vi "Ramp Wave Generator LUT.vi"(0 "frequency (periods/tick)":fxp<+,32,0>=0.0002500000409781933, 1 "reset":bool, 5 "phase offset (periods)":fxp<+,32,0>) -> (4 "saw out":i16)   [LabVIEW 2015]
doc: "Generates a point-by-point triangle wave using direct digital synthesis. The synthesis runs continuously from the top-level FPGA target clock to produce an accurate real-time frequency. Each execution of this VI returns the most recent sample produced by the underlying synthesis engine."
uses:
  <vilib>/rvi/Analysis/common/FxpNativeNode/niFpgaFxpNative.xnode
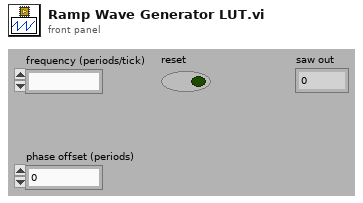
[diagram p1: front panel]
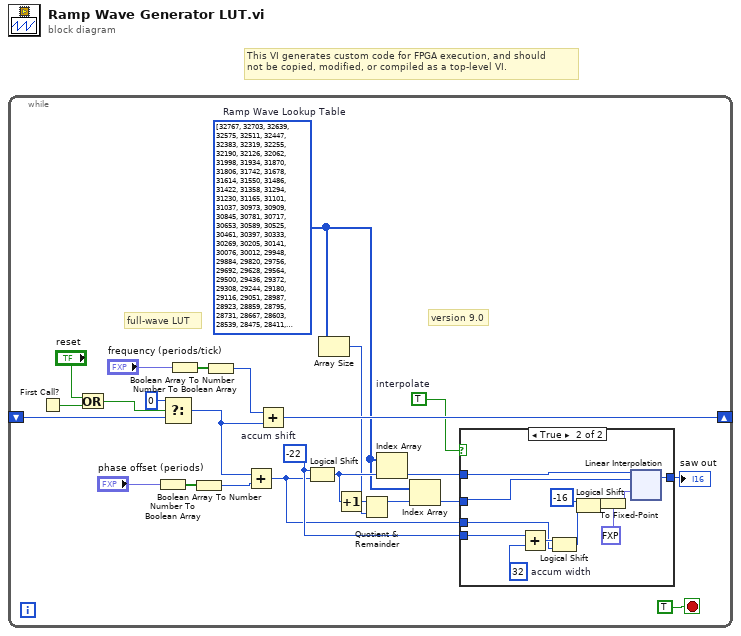
[diagram p0: block diagram]
diagram:
  # "This VI generates custom code for FPGA execution, and should\nnot be copied, modified, or compiled as a top-level VI."
  n1 = while {
    shift-right: [w24] -> _
    shift-left: _ -> [w17]
    stop <- TRUE stop-if-true
    w1 = i16[] [32767, 32703, 32639, 32575, 32511, 32447, 32383, 32319, 32255, 32190, 32126, 32062, 31998, 31934, 31870, 31806, 31742, 31678, 31614, 31550, 31486, 31422, 31358, 31294, 31230, 31165, 31101, 31037, 30973, 30909, 30845, 30781, 30717, 30653, 30589, 30525, 30461, 30397, 30333, 30269, 30205, 30141, 30076, 30012, 29948, 29884, 29820, 29756, 29692, 29628, 29564, 29500, 29436, 29372, 29308, 29244, 29180, 29116, 29051, 28987, 28923, 28859, 28795, 28731, 28667, 28603, 28539, 28475, 28411, 28347, 28283, 28219, 28155, 28091, 28027, 27962, 27898, 27834, 27770, 27706, 27642, 27578, 27514, 27450, 27386, 27322, 27258, 27194, 27130, 27066, 27002, 26937, 26873, 26809, 26745, 26681, 26617, 26553, 26489, 26425, 26361, 26297, 26233, 26169, 26105, 26041, 25977, 25913, 25848, 25784, 25720, 25656, 25592, 25528, 25464, 25400, 25336, 25272, 25208, 25144, 25080, 25016, 24952, 24888, 24823, 24759, 24695, 24631, 24567, 24503, 24439, 24375, 24311, 24247, 24183, 24119, 24055, 23991, 23927, 23863, 23799, 23734, 23670, 23606, 23542, 23478, 23414, 23350, 23286, 23222, 23158, 23094, 23030, 22966, 22902, 22838, 22774, 22709, 22645, 22581, 22517, 22453, 22389, 22325, 22261, 22197, 22133, 22069, 22005, 21941, 21877, 21813, 21749, 21685, 21620, 21556, 21492, 21428, 21364, 21300, 21236, 21172, 21108, 21044, 20980, 20916, 20852, 20788, 20724, 20660, 20595, 20531, 20467, 20403, 20339, 20275, 20211, 20147, 20083, 20019, 19955, 19891, 19827, 19763, 19699, 19635, 19571, 19506, 19442, 19378, 19314, 19250, 19186, 19122, 19058, 18994, 18930, 18866, 18802, 18738, 18674, 18610, 18546, 18481, 18417, 18353, 18289, 18225, 18161, 18097, 18033, 17969, 17905, 17841, 17777, 17713, 17649, 17585, 17521, 17457, 17392, 17328, 17264, 17200, 17136, 17072, 17008, 16944, 16880, 16816, 16752, 16688, 16624, 16560, 16496, 16432, 16367, 16303, 16239, 16175, 16111, 16047, 15983, 15919, 15855, 15791, 15727, 15663, 15599, 15535, 15471, 15407, 15343, 15278, 15214, 15150, 15086, 15022, 14958, 14894, 14830, 14766, 14702, 14638, 14574, 14510, 14446, 14382, 14318, 14253, 14189, 14125, 14061, 13997, 13933, 13869, 13805, 13741, 13677, 13613, 13549, 13485, 13421, 13357, 13293, 13229, 13164, 13100, 13036, 12972, 12908, 12844, 12780, 12716, 12652, 12588, 12524, 12460, 12396, 12332, 12268, 12204, 12139, 12075, 12011, 11947, 11883, 11819, 11755, 11691, 11627, 11563, 11499, 11435, 11371, 11307, 11243, 11179, 11115, 11050, 10986, 10922, 10858, 10794, 10730, 10666, 10602, 10538, 10474, 10410, 10346, 10282, 10218, 10154, 10090, 10025, 9961, 9897, 9833, 9769, 9705, 9641, 9577, 9513, 9449, 9385, 9321, 9257, 9193, 9129, 9065, 9001, 8936, 8872, 8808, 8744, 8680, 8616, 8552, 8488, 8424, 8360, 8296, 8232, 8168, 8104, 8040, 7976, 7911, 7847, 7783, 7719, 7655, 7591, 7527, 7463, 7399, 7335, 7271, 7207, 7143, 7079, 7015, 6951, 6887, 6822, 6758, 6694, 6630, 6566, 6502, 6438, 6374, 6310, 6246, 6182, 6118, 6054, 5990, 5926, 5862, 5797, 5733, 5669, 5605, 5541, 5477, 5413, 5349, 5285, 5221, 5157, 5093, 5029, 4965, 4901, 4837, 4773, 4708, 4644, 4580, 4516, 4452, 4388, 4324, 4260, 4196, 4132, 4068, 4004, 3940, 3876, 3812, 3748, 3683, 3619, 3555, 3491, 3427, 3363, 3299, 3235, 3171, 3107, 3043, 2979, 2915, 2851, 2787, 2723, 2659, 2594, 2530, 2466, 2402, 2338, 2274, 2210, 2146, 2082, 2018, 1954, 1890, 1826, 1762, 1698, 1634, 1569, 1505, 1441, 1377, 1313, 1249, 1185, 1121, 1057, 993, 929, 865, 801, 737, 673, 609, 545, 480, 416, 352, 288, 224, 160, 96, 32, -32, -96, -160, -224, -288, -352, -416, -480, -545, -609, -673, -737, -801, -865, -929, -993, -1057, -1121, -1185, -1249, -1313, -1377, -1441, -1505, -1569, -1634, -1698, -1762, -1826, -1890, -1954, -2018, -2082, -2146, -2210, -2274, -2338, -2402, -2466, -2530, -2594, -2659, -2723, -2787, -2851, -2915, -2979, -3043, -3107, -3171, -3235, -3299, -3363, -3427, -3491, -3555, -3619, -3683, -3748, -3812, -3876, -3940, -4004, -4068, -4132, -4196, -4260, -4324, -4388, -4452, -4516, -4580, -4644, -4708, -4773, -4837, -4901, -4965, -5029, -5093, -5157, -5221, -5285, -5349, -5413, -5477, -5541, -5605, -5669, -5733, -5797, -5862, -5926, -5990, -6054, -6118, -6182, -6246, -6310, -6374, -6438, -6502, -6566, -6630, -6694, -6758, -6822, -6887, -6951, -7015, -7079, -7143, -7207, -7271, -7335, -7399, -7463, -7527, -7591, -7655, -7719, -7783, -7847, -7911, -7976, -8040, -8104, -8168, -8232, -8296, -8360, -8424, -8488, -8552, -8616, -8680, -8744, -8808, -8872, -8936, -9001, -9065, -9129, -9193, -9257, -9321, -9385, -9449, -9513, -9577, -9641, -9705, -9769, -9833, -9897, -9961, -10025, -10090, -10154, -10218, -10282, -10346, -10410, -10474, -10538, -10602, -10666, -10730, -10794, -10858, -10922, -10986, -11050, -11115, -11179, -11243, -11307, -11371, -11435, -11499, -11563, -11627, -11691, -11755, -11819, -11883, -11947, -12011, -12075, -12139, -12204, -12268, -12332, -12396, -12460, -12524, -12588, -12652, -12716, -12780, -12844, -12908, -12972, -13036, -13100, -13164, -13229, -13293, -13357, -13421, -13485, -13549, -13613, -13677, -13741, -13805, -13869, -13933, -13997, -14061, -14125, -14189, -14253, -14318, -14382, -14446, -14510, -14574, -14638, -14702, -14766, -14830, -14894, -14958, -15022, -15086, -15150, -15214, -15278, -15343, -15407, -15471, -15535, -15599, -15663, -15727, -15791, -15855, -15919, -15983, -16047, -16111, -16175, -16239, -16303, -16367, -16432, -16496, -16560, -16624, -16688, -16752, -16816, -16880, -16944, -17008, -17072, -17136, -17200, -17264, -17328, -17392, -17457, -17521, -17585, -17649, -17713, -17777, -17841, -17905, -17969, -18033, -18097, -18161, -18225, -18289, -18353, -18417, -18481, -18546, -18610, -18674, -18738, -18802, -18866, -18930, -18994, -19058, -19122, -19186, -19250, -19314, -19378, -19442, -19506, -19571, -19635, -19699, -19763, -19827, -19891, -19955, -20019, -20083, -20147, -20211, -20275, -20339, -20403, -20467, -20531, -20595, -20660, -20724, -20788, -20852, -20916, -20980, -21044, -21108, -21172, -21236, -21300, -21364, -21428, -21492, -21556, -21620, -21685, -21749, -21813, -21877, -21941, -22005, -22069, -22133, -22197, -22261, -22325, -22389, -22453, -22517, -22581, -22645, -22709, -22774, -22838, -22902, -22966, -23030, -23094, -23158, -23222, -23286, -23350, -23414, -23478, -23542, -23606, -23670, -23734, -23799, -23863, -23927, -23991, -24055, -24119, -24183, -24247, -24311, -24375, -24439, -24503, -24567, -24631, -24695, -24759, -24823, -24888, -24952, -25016, -25080, -25144, -25208, -25272, -25336, -25400, -25464, -25528, -25592, -25656, -25720, -25784, -25848, -25913, -25977, -26041, -26105, -26169, -26233, -26297, -26361, -26425, -26489, -26553, -26617, -26681, -26745, -26809, -26873, -26937, -27002, -27066, -27130, -27194, -27258, -27322, -27386, -27450, -27514, -27578, -27642, -27706, -27770, -27834, -27898, -27962, -28027, -28091, -28155, -28219, -28283, -28347, -28411, -28475, -28539, -28603, -28667, -28731, -28795, -28859, -28923, -28987, -29051, -29116, -29180, -29244, -29308, -29372, -29436, -29500, -29564, -29628, -29692, -29756, -29820, -29884, -29948, -30012, -30076, -30141, -30205, -30269, -30333, -30397, -30461, -30525, -30589, -30653, -30717, -30781, -30845, -30909, -30973, -31037, -31101, -31165, -31230, -31294, -31358, -31422, -31486, -31550, -31614, -31678, -31742, -31806, -31870, -31934, -31998, -32062, -32126, -32190, -32255, -32319, -32383, -32447, -32511, -32575, -32639, -32703, -32767]  # Ramp Wave Lookup Table
    w20 = TRUE  # interpolate
    w19 = i8 -22  # accum shift
    # "version 9.0"
    # "full-wave LUT"
    n2 = First Call?() -> (First Call?: T/F=w15:bool)
    n3 = Or(x="reset", y=w15) -> (x .or. y?=w14:bool)
    n4 = Number To Boolean Array(number="phase offset (periods)") -> (Boolean array=w4:bool[])
    n5 = Select(t=u32 0, s=w14, f=w17) -> (s? t:f=w22:u32)
    n6 = Number To Boolean Array(number="frequency (periods/tick)") -> (Boolean array=w7:bool[])
    n7 = Boolean Array To Number(Boolean array=w4) -> (number=w2:u32)
    n8 = Boolean Array To Number(Boolean array=w7) -> (number=w5:u32)
    n9 = Add(x=w22, y=w2) -> (x+y=w18:u32)
    n10 = Add(x=w5, y=w22) -> (x+y=w24:u32)
    n11 = Logical Shift(y=w19, x=w18) -> (x << y=w12:u32)
    n12 = Array Size(array=w1) -> (size(s)=w8:i32)
    n13 = Increment(x=w12) -> (x+1=w13:u32)
    n14 = Quotient & Remainder(x=w13, y=w8) -> (x-y*floor(x/y)=w10:u32)  [unwired: 1 out]
    n15 = Index Array(array=w1, index=w12) -> (element=w11:i16)
    n16 = Index Array(array=w1, index=w10) -> (element=w9:i16)
    n17 = case shown="True" w20 {
      tunnel: w11 -> [w26 w29]
      tunnel: [w26 w28] -> w21
      tunnel: w19 -> [_ w38]
      tunnel: w18 -> [_ w35]
      tunnel: w9 -> [_ w30]
      frame False {
      }
      frame True {
        w37 = i8 32  # accum width
        n18 = Add(x=w38, y=w37) -> (x+y=w36:i8)
        n19 = Logical Shift(y=w36, x=w35) -> (x << y=w34:u32)
        n20 = Logical Shift(y=-16, x=w34) -> (x << y=w32:u32)
        n21 = To Fixed-Point(fixed-point type=fxp<+,16,0> 0.0, number=w32) -> (fixed-point=w31:fxp<+,16,0>)
        n22 = xnode ("Linear Interpolation")("y0"=w29, "y1"=w30, "x"=w31) -> ("y"=w28:i16)
      }
    }
    "saw out" <- w21
  }
